vi "TEST LVOOP Plug Ins.vi"(8 "error in (no error)":errorcluster, 10 "Queue Name":string="Main") -> (0 "error out":errorcluster)   [LabVIEW 2011]
doc: "This stub VI is provided in the LVOOP Plug Ins exercise. Minimal and simple modifications to the code are required to implement Plug Ins for LVOOP.\n\nAAL 9/09"
uses:
  Shared/QDMH Poly VIs/QDMH POLY Enqueue String.vi
  Shared/QDMH Poly VIs/QDMH POLY Enqueue Strings.vi
  Report Class/Report.lvclass
panel:
  in  "Get Plug Ins":bool
  in  "File Name (no extension)":string
  in  "Header":string
  in  "Save to File":bool
  in  "Available Plug Ins":u16(ring) items=["TXT_Report", "XML Report"]
  out "Message Display":string
  in  "Cancel":bool
  in  "OK":bool
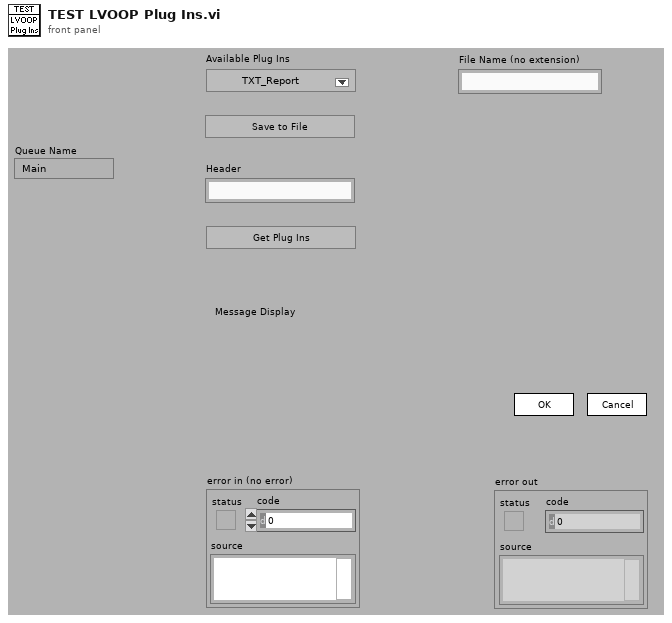
[diagram p1: front panel]
types:
  T1 = cluster{"Operator Name":string, "Current VI's Path":path, "Queue Names":string[], "# VIs Launched":i32, "Report Objects":refnum<class "Report.lvclass">[], "Selected Plug In":i32, "Current VI's Directory":path}
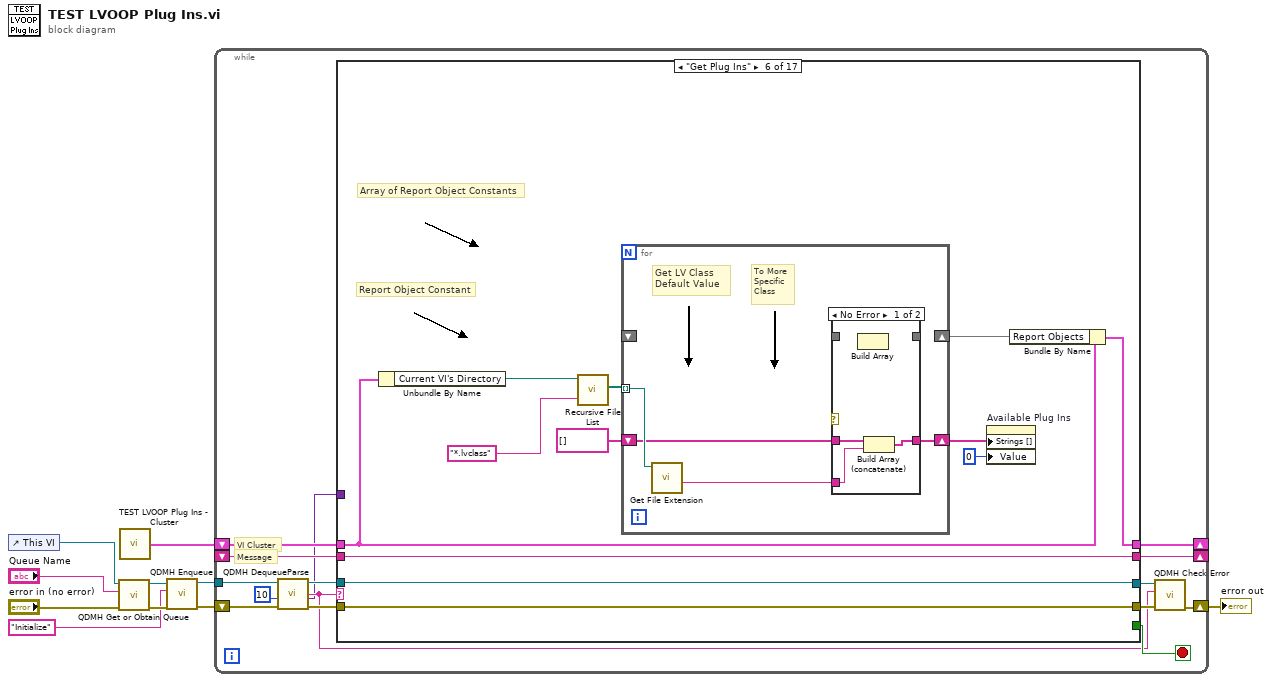
[diagram p0: block diagram]
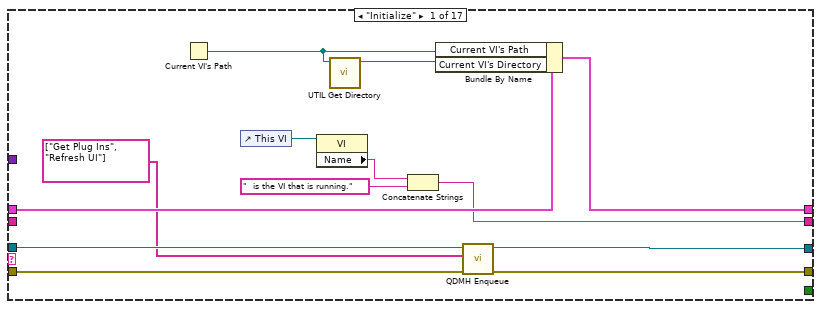
[diagram p2: hidden frame]
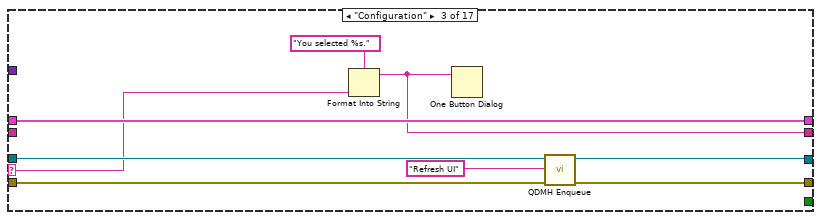
[diagram p4: hidden frame]
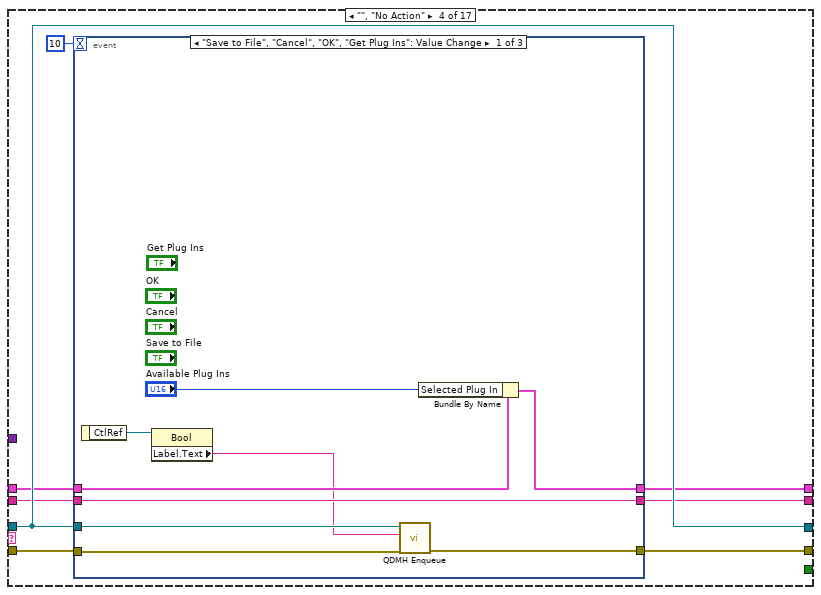
[diagram p5: hidden frame]
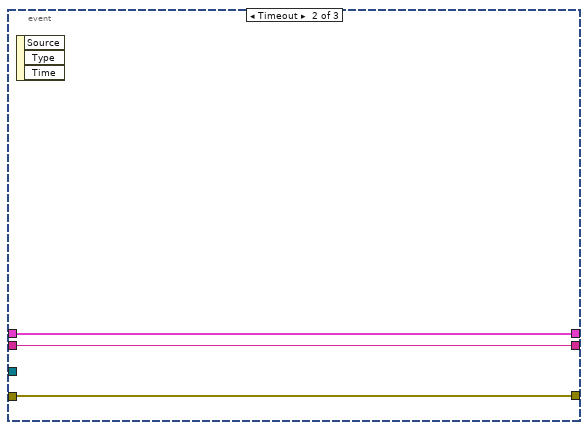
[diagram p6: hidden frame]
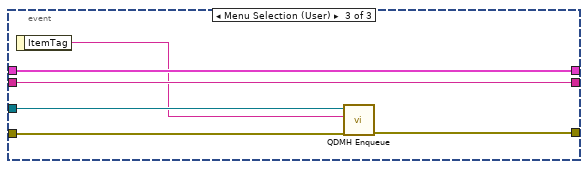
[diagram p7: hidden frame]
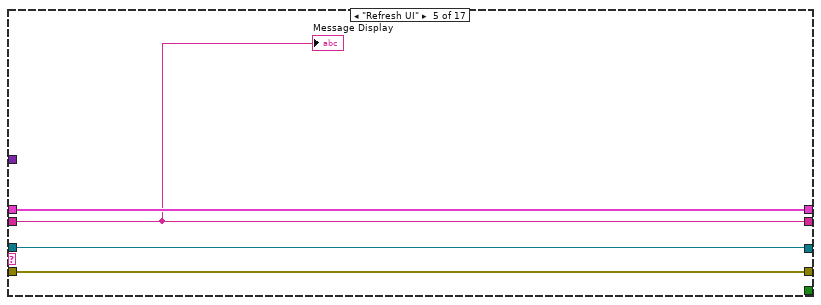
[diagram p8: hidden frame]
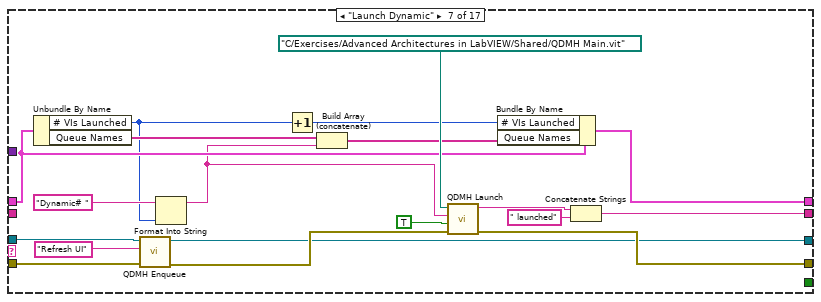
[diagram p10: hidden frame]
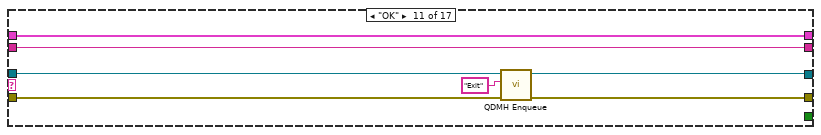
[diagram p14: hidden frame]
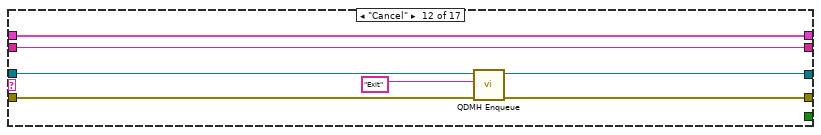
[diagram p15: hidden frame]
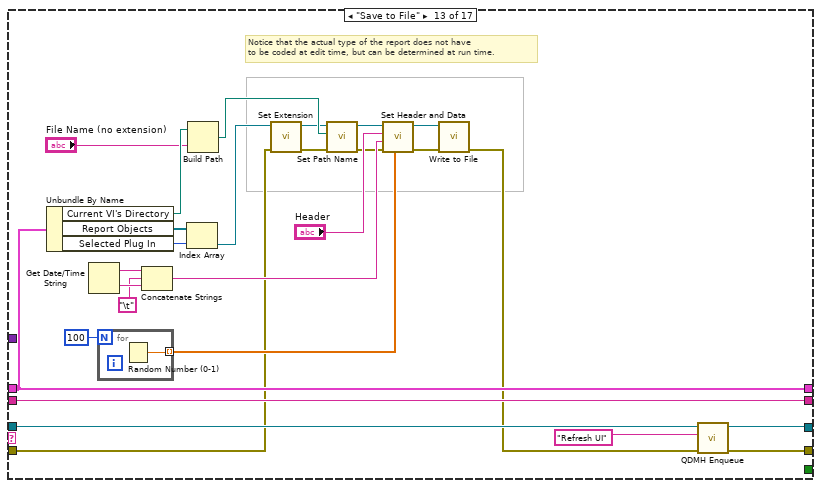
[diagram p16: hidden frame]
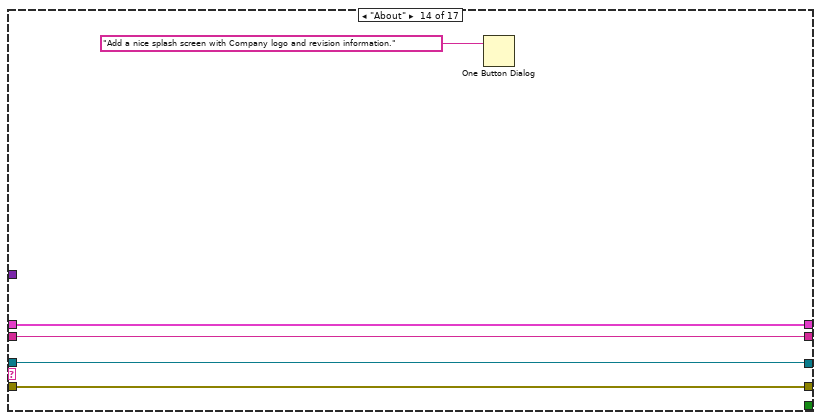
[diagram p17: hidden frame]
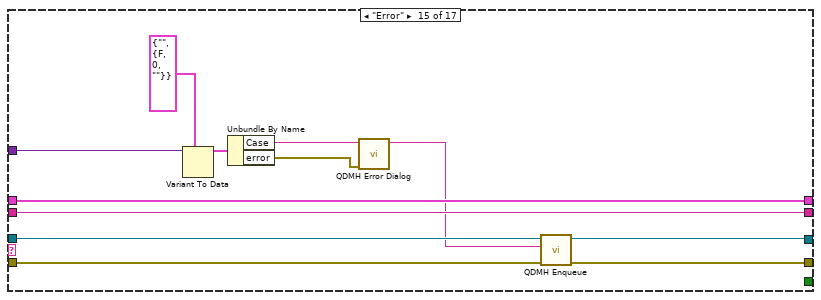
[diagram p18: hidden frame]
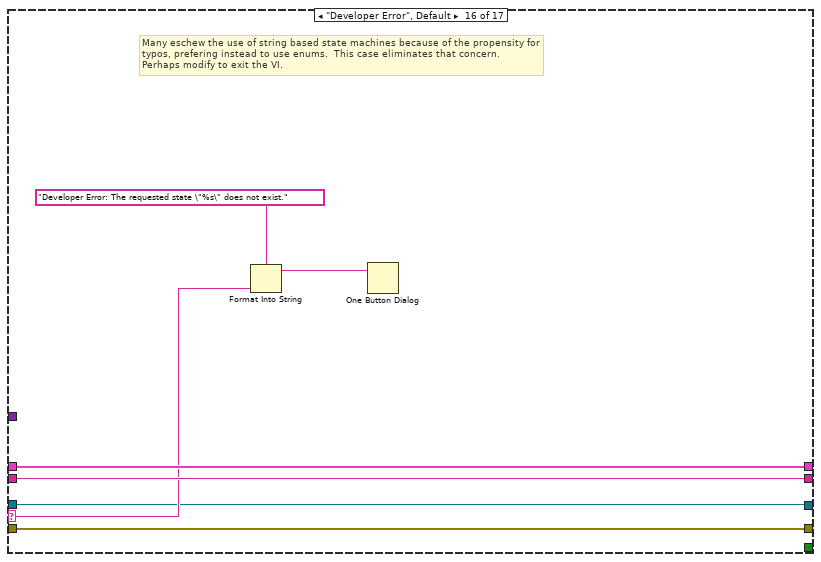
[diagram p19: hidden frame]
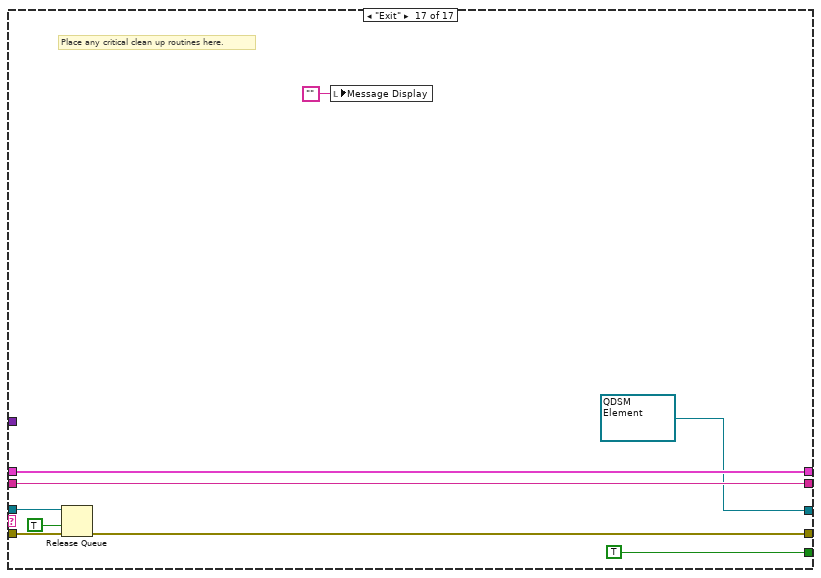
[diagram p20: hidden frame]
diagram:
  n1 = control-ref of="This VI"() -> (w2:refnum<vi>)
  n2 = call "QDMH Get or Obtain Queue.vi"("error in (no error)"="error in (no error)", "Queue Name"="Queue Name", "VI Refnum"=w2) -> ("error out"=w6:errorcluster, "queue out"=w9:refnum<queue>)  [unwired: 7 out]
  n3 = call "TEST LVOOP Plug Ins - Cluster.vi"() -> ("Cluster"=w8:T1)
  n4 = call-poly "QDMH Enqueue.vi"("error in (no error)"=w6, "State"="Initialize" ("element"), "queue"=w9) -> ("error out"=w7:errorcluster, "queue out"=w10:refnum<queue>)  [unwired: 7 in]
  n5 = while {
    tunnel: w10 -> [w21]
    shift-left: w8 -> [w22]
    shift-right: [w23] -> _
    shift-left: _ -> [w24]
    shift-right: [w14] -> _
    shift-right: [w12] -> w4
    shift-left: w7 -> [w17]
    stop <- w25 stop-if-true
    # "VI Cluster"
    # "Message"
    n6 = call "QDMH DequeueParse.vi"("error in (no error)"=w17, "Timeout"=10 ("ms timeout (-1)"), "queue"=w21) -> ("error out"=w18:errorcluster, "Variant Data"=w11:variant, "State"=w13:string, "queue out"=w19:refnum<queue>)  [unwired: 5 out]
    n7 = case shown="\"Get Plug Ins\"" w13 {
      selector: w13 -> [_ _ w47 _ _ _ _ _ _ _ _ _ _ _ _ w196 _]
      tunnel: w19 -> [w31 w39 w49 w59 w78 w82 w116 w122 w126 w130 w140 w147 w174 w176 w190 w193 w205]
      tunnel: [_ _ _ _ _ _ _ _ _ _ _ _ _ _ _ _ TRUE] -> w25
      tunnel: [w35 w42 w48 w52 w80 w93 w117 w125 w129 w133 w139 w146 w173 w180 w192 w199 w207] -> w14
      tunnel: w24 -> [_ w42 _ w53 w80 w93 _ w125 w129 w133 w139 w146 w173 w180 w192 w199 w207]
      tunnel: [w37 w41 w51 w54 w81 w90 w113 w124 w128 w132 w138 w145 w171 w179 w191 w198 w202] -> w23
      tunnel: w22 -> [w38 w41 w51 w55 w81 w91 w114 w124 w128 w132 w138 w145 w171 w179 w191 w198 w202]
      tunnel: w18 -> [w32 w40 w46 w58 w79 w92 w107 w123 w127 w131 w137 w144 w152 w177 w189 w195 w204]
      tunnel: [w28 w40 w45 w57 w79 w92 w106 w123 w127 w131 w136 w143 w172 w177 w188 w195 w201] -> w16
      tunnel: [w27 w39 w43 w59 w78 w82 w103 w122 w126 w130 w134 w142 w162 w176 w187 w193 refnum<queue> refnum ("queue out")] -> w15
      tunnel: w11 -> [_ _ _ _ _ _ _ _ _ _ _ _ _ _ w182 _ _]
      frame "Initialize" {
        n8 = Current VI's Path() -> (path=w30:path)
        n9 = control-ref of="This VI"() -> (w34:refnum<vi>)
        n10 = property class="VI"(reference=w34) -> ("Name"=w33:string)  [unwired: 1 in, 2 out]
        n11 = call "UTIL Get Directory.vi"("Path In"=w30) -> ("Directory Out"=w29:path)  [unwired: 1 in, 9 out]
        n12 = Concatenate Strings(w33, "  is the VI that is running." ("string")) -> (w35:string)
        n13 = Bundle By Name(cluster=w38, "Current VI's Path"=w30, "Current VI's Directory"=w29) -> (w37:T1)
        n14 = call-poly "QDMH Enqueue.vi"("error in (no error)"=w32, "States"=string[] ["Get Plug Ins", "Refresh UI"], "queue"=w31) -> ("error out"=w28:errorcluster, "queue out"=w27:refnum<queue>)  [unwired: 7 in]
      }
      frame "Re-Initialize" {
        # "This case includes initialization functionality that may need to run again during the course of the VI"
      }
      frame "Configuration" {
        n15 = Format Into String(format string="You selected %s." ("Format String"), w47) -> (resulting string=w48:string)  [unwired: 2 in, 1 out]
        n16 = One Button Dialog(message=w48) -> ()  [unwired: 2 out]
        n17 = call-poly "QDMH Enqueue.vi"("error in (no error)"=w46, "State"="Refresh UI" ("New State"), "queue"=w49) -> ("error out"=w45:errorcluster, "queue out"=w43:refnum<queue>)  [unwired: 7 in]
      }
      frame "", "No Action" {
        n18 = event shown="[0] \"Save to File\", \"Cancel\", \"OK\", \"Get Plug Ins\": Value Change" {
          selector: _ -> [_ _ _]
          dyn-events: _ -> [_ _ _]
          timeout: 10 -> [_ _ _]
          tunnel: w59 -> [w67 _ w77]
          tunnel: [w66 w71 w75] -> w57
          tunnel: w58 -> [w65 w71 w76]
          tunnel: w55 -> [w63 w70 w74]
          tunnel: [w62 w70 w74] -> w54
          tunnel: w53 -> [w64 w69 w73]
          tunnel: [w64 w69 w73] -> w52
          event "Save to File", "Cancel", "OK", "Get Plug Ins": Value Change {
            n19 = event-data() -> ("CtlRef"=w68:refnum<vi>)  [unwired: 1 out]
            n20 = property class="Bool"(reference=w68) -> ("Label.Text"=w60:string)  [unwired: 1 in, 2 out]
            n21 = call-poly "QDMH Enqueue.vi"("error in (no error)"=w65, "State"=w60, "queue"=w67) -> ("error out"=w66:errorcluster)  [unwired: 7 in, 1 out]
            n22 = Bundle By Name(cluster=w63, "Selected Plug In"="Available Plug Ins") -> (w62:T1)
          }
          event Timeout {
            n23 = event-data() -> ()  [unwired: 4 out]
          }
          event Menu Selection (User) {
            n24 = event-data() -> ("ItemTag"=w72:string)  [unwired: 1 out]
            n25 = call-poly "QDMH Enqueue.vi"("error in (no error)"=w76, "State"=w72, "queue"=w77) -> ("error out"=w75:errorcluster)  [unwired: 7 in, 1 out]
          }
        }
      }
      frame "Refresh UI" {
        "Message Display" <- w80
      }
      frame "Get Plug Ins" {
        # "Array of Report Object Constants"
        # "Report Object Constant"
        n26 = Unbundle By Name(w91) -> ("Current VI's Directory"=w83:path)
        n27 = call <vilib>:"Recursive File List.vi"("pattern"="*.lvclass", "Folder Path"=w83) -> ("All Files in Dir"=w87:path[])  [unwired: 2 in, 7 out]
        n28 = for {
          tunnel: w87 -> [w97] mode=indexing
          shift-right: [_] -> w86
          shift-left: _ -> [_]
          shift-right: [w95] -> w85
          shift-left: string[] [] -> [w96]
          # "To More\nSpecific\nClass"
          # "Get LV Class Default Value"
          n29 = call <vilib>:"Get File Extension.vi"("file"=w97) -> ("filename without extension"=w94:string)  [unwired: 1 in, 9 out]
          n30 = case shown="No Error" {
            selector: _ -> [_ _]
            tunnel: _ -> [_ w102]
            tunnel: [_ w102] -> _
            tunnel: w96 -> [w100 w101]
            tunnel: [w99 w101] -> w95
            tunnel: w94 -> [w98 _]
            frame No Error {
              n31 = Build Array() -> ()  [unwired: 2 in, 1 out]
              n32 = Build Array (concatenate)(w100, w98) -> (w99:string[])
            }
            frame Error {
            }
          }
        }
        n33 = property on="Available Plug Ins" class="Ring (strict)"("Strings []"=w85, "Value"=0) -> ()  [unwired: 2 in, 2 out]
        n34 = Bundle By Name(cluster=w91, "Report Objects"=w86) -> (w90:T1)
      }
      frame "Launch Dynamic" {
        n35 = Unbundle By Name(w114) -> ("# VIs Launched"=w110:i32, "Queue Names"=w112:string[])
        n36 = call-poly "QDMH Enqueue.vi"("error in (no error)"=w107, "State"="Refresh UI" ("New State"), "queue"=w116) -> ("error out"=w104:errorcluster, "queue out"=w103:refnum<queue>)  [unwired: 7 in]
        n37 = Format Into String(initial string="Dynamic# ", w110) -> (resulting string=w108:string)  [unwired: 2 in, 1 out]
        n38 = Increment(x=w110) -> (x+1=w109:i32)
        n39 = Build Array (concatenate)(w112, w108) -> (w111:string[])
        n40 = call "QDMH Launch.vi"("error in (no error)"=w104, "Front Panel Window (Open)"=TRUE ("Front Panel Window:Open"), "Queue Name"=w108, "VI Path"=path "C:/Exercises/Advanced Architectures in LabVIEW/Shared/QDMH Main.vit" ("vi path")) -> ("error out"=w106:errorcluster, "Launched VI Name"=w119:string)  [unwired: 6 out]
        n41 = Bundle By Name(cluster=w114, "# VIs Launched"=w109, "Queue Names"=w111) -> (w113:T1)
        n42 = Concatenate Strings(w119, " launched" ("string")) -> (w117:string)
      }
      frame "Shutdown Dynamic" {
      }
      frame "Send Message to Dynamic" {
      }
      frame "Receive Message From Dynamic" {
      }
      frame "OK" {
        n43 = call-poly "QDMH Enqueue.vi"("error in (no error)"=w137, "State"="Exit" ("New State"), "queue"=w140) -> ("error out"=w136:errorcluster, "queue out"=w134:refnum<queue>)  [unwired: 7 in]
      }
      frame "Cancel" {
        n44 = call-poly "QDMH Enqueue.vi"("error in (no error)"=w144, "State"="Exit" ("New State"), "queue"=w147) -> ("error out"=w143:errorcluster, "queue out"=w142:refnum<queue>)  [unwired: 7 in]
      }
      frame "Save to File" {
        # "Notice that the actual type of the report does not have\nto be coded at edit time, but can be determined at run time."
        n45 = Unbundle By Name(w171) -> ("Current VI's Directory"=w164:path, "Report Objects"=w169:refnum<class "Report.lvclass">[], "Selected Plug In"=w170:i32)
        n46 = Get Date/Time String() -> (date string=w166:string, time string=w168:string)  [unwired: 3 out]
        n47 = for {
          N: 100 -> [_]
          tunnel: [w175] -> w155 mode=indexing
          n48 = Random Number (0-1)() -> (number: 0 to 1=w175:dbl)
        }
        n49 = Concatenate Strings(w166, "\t", w168) -> (w153:string)
        n50 = Index Array(array=w169, index=w170) -> (element=w159:refnum<class "Report.lvclass">)
        n51 = Build Path(base path=w164, name or relative path="File Name (no extension)") -> (appended path=w160:path)
        n52 = call-dynamic "Set Extension.vi"("error in (no error)"=w152, "Report"=w159) -> ("error out"=w151:errorcluster, "Report out"=w158:refnum<class "Report.lvclass">)  [unwired: 8 in]
        n53 = call-dynamic "Set Path Name.vi"("error in (no error)"=w151, "Path"=w160, "Report"=w158) -> ("error out"=w150:errorcluster, "Report out"=w157:refnum<class "Report.lvclass">)  [unwired: 7 in]
        n54 = call-dynamic "Set Header and Data.vi"("Data Array"=w155, "error in (no error)"=w150, "Data & Time String"=w153, "Header"="Header", "Report"=w157) -> ("error out"=w149:errorcluster, "Report out"=w156:refnum<class "Report.lvclass">)  [unwired: 5 in]
        n55 = call-dynamic "Write to File.vi"("error in (no error)"=w149, "Report"=w156) -> ("error out"=w148:errorcluster)  [unwired: 8 in, 1 out]
        n56 = call-poly "QDMH Enqueue.vi"("error in (no error)"=w148, "State"="Refresh UI" ("New State"), "queue"=w174) -> ("error out"=w172:errorcluster, "queue out"=w162:refnum<queue>)  [unwired: 7 in]
      }
      frame "About" {
        n57 = One Button Dialog(message="Add a nice splash screen with Company logo and revision information.") -> ()  [unwired: 2 out]
      }
      frame "Error" {
        n58 = Variant To Data(type=cluster{"Case":string, "error":errorcluster} {"Case"="", "error"={"status"=FALSE, "code"=0, "source"=""}} ("QDSM Element"), Variant=w182) -> (data=w185:cluster{"Case":string, "error":errorcluster})  [unwired: 1 in, 1 out]
        n59 = Unbundle By Name(w185) -> ("Case"=w184:string, "error"=w183:errorcluster)
        n60 = call "QDMH Error Dialog.vi"("error"=w183, "Case Error Occured"=w184) -> ("Case to Execute"=w181:string)  [unwired: 9 out]
        n61 = call-poly "QDMH Enqueue.vi"("error in (no error)"=w189, "State"=w181, "queue"=w190) -> ("error out"=w188:errorcluster, "queue out"=w187:refnum<queue>)  [unwired: 7 in]
      }
      frame "Developer Error", Default {
        # "Many eschew the use of string based state machines because of the propensity for\ntypos, prefering instead to use enums.  This case eliminates that concern.\nPerhaps modify to exit the VI."
        n62 = Format Into String(format string="Developer Error: The requested state \"%s\" does not exist." ("message"), w196) -> (resulting string=w194:string)  [unwired: 2 in, 1 out]
        n63 = One Button Dialog(message=w194) -> ()  [unwired: 2 out]
      }
      frame "Exit" {
        # "Place any critical clean up routines here."
        n64 = Release Queue(queue=w205, force destroy? (F)=TRUE, error in (no error)=w204) -> (error out=w201:errorcluster)  [unwired: 2 out]
        n65 = local write "Message Display"("") -> ()
      }
    }
    n66 = call "QDMH Check Error.vi"("error in (no error)"=w16, "Case"=w13, "queue"=w15) -> ("error out"=w12:errorcluster)  [unwired: 7 in, 1 out]
  }
  "error out" <- w4
